vi "Wait for Process.vi"(8 "error in":errorcluster, 11 "Process Executor in":refnum<class "Process Executor.lvclass">) -> (0 "error out":errorcluster, 3 "Process Executor out":refnum<class "Process Executor.lvclass">)   [LabVIEW 2025, in "Process Executor.lvclass"]
doc: "Waits for a process to complete, optionally enforcing a timeout. If the timeout is >0 the VI waits for the specified seconds for the process to complete. If a timeout occurs, an error is produced. If the timeout is <0, the VI waits indefinitely for the process to complete. If the timeout is 0 the VI exits immediately, letting the process run in the background (fire and forget)."
uses:
  Process Executor.lvclass
  Process Executor.lvclass/Process Executor.ctl
  C:/Program Files (x86)/dotnet/shared/Microsoft.NETCore.App/8.0.23/System.Diagnostics.Process.dll
  Program Files (x86)/dotnet/shared/Microsoft.NETCore.App/8.0.23/System.Diagnostics.Process.dll
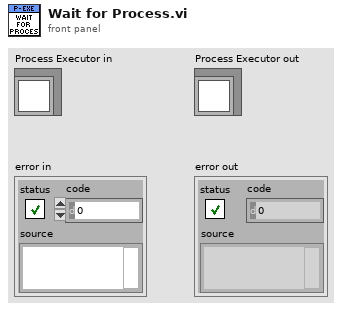
[diagram p1: front panel]
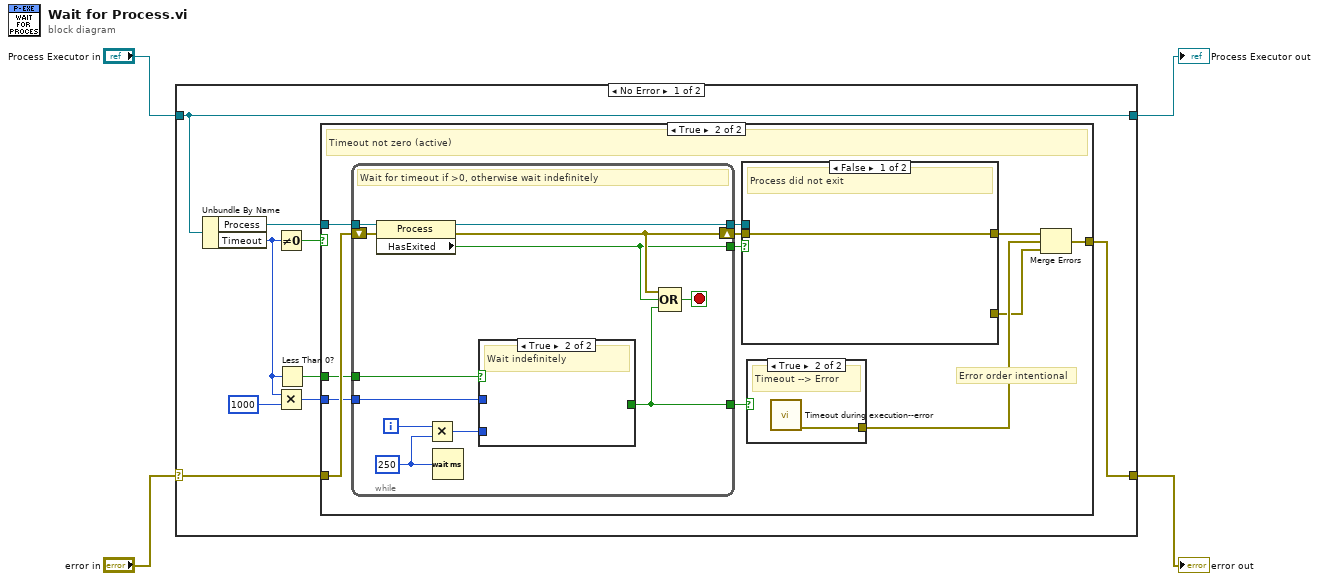
[diagram p0: block diagram]
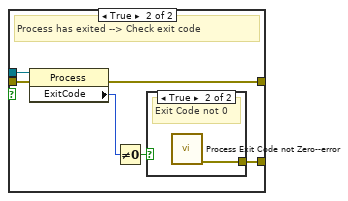
[diagram p3: hidden frame]
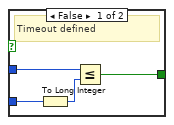
[diagram p6: hidden frame]
diagram:
  n1 = case shown="No Error" "error in" {
    selector: "error in" -> [w13 w52]
    tunnel: [w12 w52] -> w3
    tunnel: [w11 w51] -> w1
    tunnel: "Process Executor in" -> [w11 w51]
    frame No Error {
      n2 = Unbundle By Name(w11) -> ("Process"=w9:refnum<k39>, "Timeout"=w5:i32)
      n3 = Not Equal To 0?(x=w5) -> (x != 0?=w6:bool)
      n4 = Multiply(x=w5, y=1000) -> (x*y=w8:i32)
      n5 = Less Than 0?(x=w5) -> (x < 0?=w7:bool)
      n6 = case shown="True" w6 {
        tunnel: w9 -> [_ w19]
        tunnel: w13 -> [_ w25]
        tunnel: w8 -> [_ w18]
        tunnel: w7 -> [_ w17]
        tunnel: [_ w23] -> w12
        frame False {
          # "Timeout = 0 --> Fire and forget"
        }
        frame True {
          # "Error order intentional"
          # "Timeout not zero (active)"
          n7 = while {
            tunnel: w19 -> [w44]
            shift-right: [w45] -> w21
            shift-left: w25 -> [w46]
            tunnel: w18 -> [w41]
            tunnel: w17 -> [w38]
            tunnel: [w37] -> w16
            tunnel: [w36] -> w15
            tunnel: [w35] -> w14
            i -> [w42]
            stop <- w39 stop-if-true
            w43 = u32 250 ("milliseconds to wait")
            # "Wait for timeout if >0, otherwise wait indefinitely"
            n8 = property on="Property Node" class="Process"(reference=w44, error in=w46) -> (reference out=w36:refnum<k39>, error out=w45:errorcluster, "HasExited"=w35:bool)
            n9 = Multiply(x=w42, y=w43) -> (x*y=w40:u32)
            n10 = Wait (ms)(milliseconds to wait=w43) -> ()  [unwired: 1 out]
            n11 = case shown="True" w38 {
              tunnel: w41 -> [w50 _]
              tunnel: w40 -> [w49 _]
              tunnel: [w47 _] -> w37
              frame False {
                # "Timeout defined"
                n12 = To Long Integer(number=w49) -> (32bit integer=w48:i32)
                n13 = Less Or Equal?(x=w50, y=w48) -> (x <= y?=w47:bool)
              }
              frame True {
                # "Wait indefinitely"
              }
            }
            n14 = Compound Arithmetic op=OR(w45, w35, w37) -> (w39:bool)
          }
          n15 = case shown="False" w14 {
            tunnel: [_ w32] -> w22
            tunnel: w21 -> [w26 w31]
            tunnel: [w26 w30] -> w20
            tunnel: w15 -> [_ w28]
            frame False {
              # "Process did not exit"
            }
            frame True {
              # "Process has exited --> Check exit code"
              n16 = property class="Process"(reference=w28, error in=w31) -> (error out=w30:errorcluster, "ExitCode"=w27:i32)  [unwired: 1 out]
              n17 = Not Equal To 0?(x=w27) -> (x != 0?=w29:bool)
              n18 = case shown="True" w29 {
                tunnel: [_ w33] -> w32
                frame False {
                  # "Exit code 0"
                }
                frame True {
                  # "Exit Code not 0"
                  n19 = call "Process Exit Code not Zero--error.vi"() -> ("error out"=w33:errorcluster)  [unwired: 11 in]
                }
              }
            }
          }
          n20 = case shown="True" w16 {
            tunnel: [_ w34] -> w24
            frame False {
              # "No timeout"
            }
            frame True {
              # "Timeout --> Error"
              n21 = call "Timeout during execution--error.vi"() -> ("error out"=w34:errorcluster)  [unwired: 11 in]
            }
          }
          n22 = Merge Errors(w20, w24, w22) -> (w23:errorcluster)
        }
      }
    }
    frame Error {
    }
  }
  "error out" <- w3
  "Process Executor out" <- w1
